vi "Connect.vi"(8 "error in (no error)":errorcluster, 11 "Postgres Connector In":refnum<class "Postgres Connector.lvclass">) -> (0 "error out":errorcluster, 3 "Postgres Connector Out":refnum<class "Postgres Connector.lvclass">)   [LabVIEW 2020, in "Postgres Connector.lvclass"]
doc: "This VI establish a connection with the server using TCP. After, it connect the user to a database.\n\nC:\\Program Files (x86)\\National Instruments\\LabVIEW 2014\\help\\Neosoft Technologies\\NeoDB for PostgreSQL\\NeoDB for PostgreSQL User Manual.pdf"
uses:
  Postgres Connector.lvclass
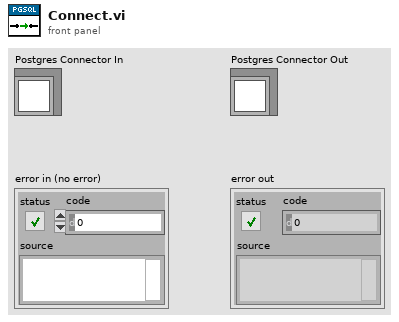
[diagram p1: front panel]
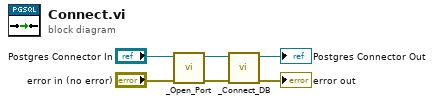
[diagram p0: block diagram]
diagram:
  n1 = call "_Open_Port.vi"("error in (no error)"="error in (no error)", "Postgres Connector.lvclass"="Postgres Connector In") -> ("error out"=w2:errorcluster, "output cluster"=w3:refnum<class "Postgres Connector.lvclass">)  [unwired: 8 in]
  n2 = call "_Connect_DB.vi"("error in (no error)"=w2, "Postgres Connector In"=w3) -> ("error out"=→"error out":errorcluster, "Postgres Connector Out"=→"Postgres Connector Out":refnum<class "Postgres Connector.lvclass">)  [unwired: 8 in]
